vi "Generate Trajectory.vi"(6 "Overrides 2":T1(array[cluster]), 7 "Stoopid Overlap %":dbl min=0.0, 8 "Conditions":T3, 9 "Limits":T2={"Velocity (fps)"=6.0, "Accel (fps^2)"=15.0, "Jerk (fps^3)"=150.0, "StoopidFast (fps)"=6.0} {"StoopidFast (fps)" min=0.0; "Jerk (fps^3)" min=0.0 step=1.0; "Accel (fps^2)" min=0.0; "Velocity (fps)" min=0.0}, 10 "WayPoints":cluster{"x":dbl, "y":dbl, "th":dbl}[](array[cluster]), 11 "Sample Period (s)":dbl=0.02) -> (0 "Updated Waypoints":cluster{"x":dbl, "y":dbl, "th":dbl}[](array[cluster]), 1 "Valid":bool, 2 "Time (s)":dbl, 3 "Trajectory Data":T4(array[cluster]), 4 "Distance (ft)":dbl)   [LabVIEW 2019]
uses:
  Limits.ctl
  Speeds.ctl
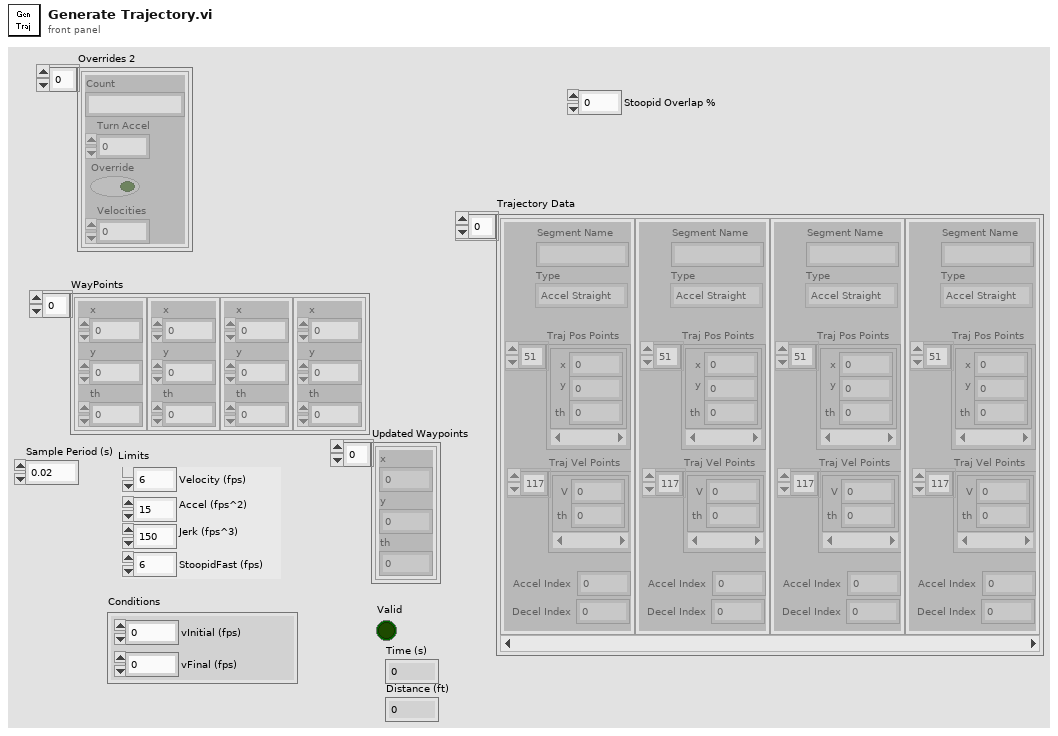
[diagram p1: front panel]
types:
  T1 = cluster{"Count":string, "Turn Accel":dbl, "Override":bool, "Velocities":dbl}[]
  T2 = typedef "Limits.ctl" = cluster{"Velocity (fps)":dbl, "Accel (fps^2)":dbl, "Jerk (fps^3)":dbl, "StoopidFast (fps)":dbl}
  T3 = cluster{"vInitial (fps)":dbl, "vFinal (fps)":dbl}
  T4 = cluster{"Segment Name":string, "Type":enum16{"Accel Straight", "Const Straight", "Blend", "Circle"}, "Traj Pos Points":cluster{"x":dbl, "y":dbl, "th":dbl}[], "Traj Vel Points":cluster{"V":dbl, "th":dbl}[], "Accel Index":i32, "Decel Index":i32}[]
  T5 = typedef "Speeds.ctl" = cluster{"maxV (fps)":dbl, "Accel Limit (fps^2)":dbl, "Initial V (fps)":dbl, "Sample Period (s)":dbl, "Jerk Limit (fps^3)":dbl, "Distances":cluster{"distance (ft)":dbl, "baseline (ft)":dbl, "high (ft)":dbl}[]}
  T6 = cluster{"Count":string, "Turn Accel":dbl, "Override":bool, "Velocities":dbl}
  T7 = cluster{"Point Out":cluster{"x":dbl, "y":dbl, "th":dbl}, "Point Out":cluster{"x":dbl, "y":dbl, "th":dbl}, "Valid":bool}[]
  T8 = typedef "BlendType.ctl" = cluster{"Scaling":dbl, "Length":dbl, "Angle":dbl, "Vertex Dist":dbl, "ParaTime":dbl, "ExtraArc":dbl, "Center Point":cluster{dbl, dbl}, "Radius":dbl}
  T9 = cluster{"Segment Name":string, "Type":enum16{"Accel Straight", "Const Straight", "Blend", "Circle"}, "Traj Pos Points":cluster{"x":dbl, "y":dbl, "th":dbl}[], "Traj Vel Points":cluster{"V":dbl, "th":dbl}[], "Accel Index":i32, "Decel Index":i32}
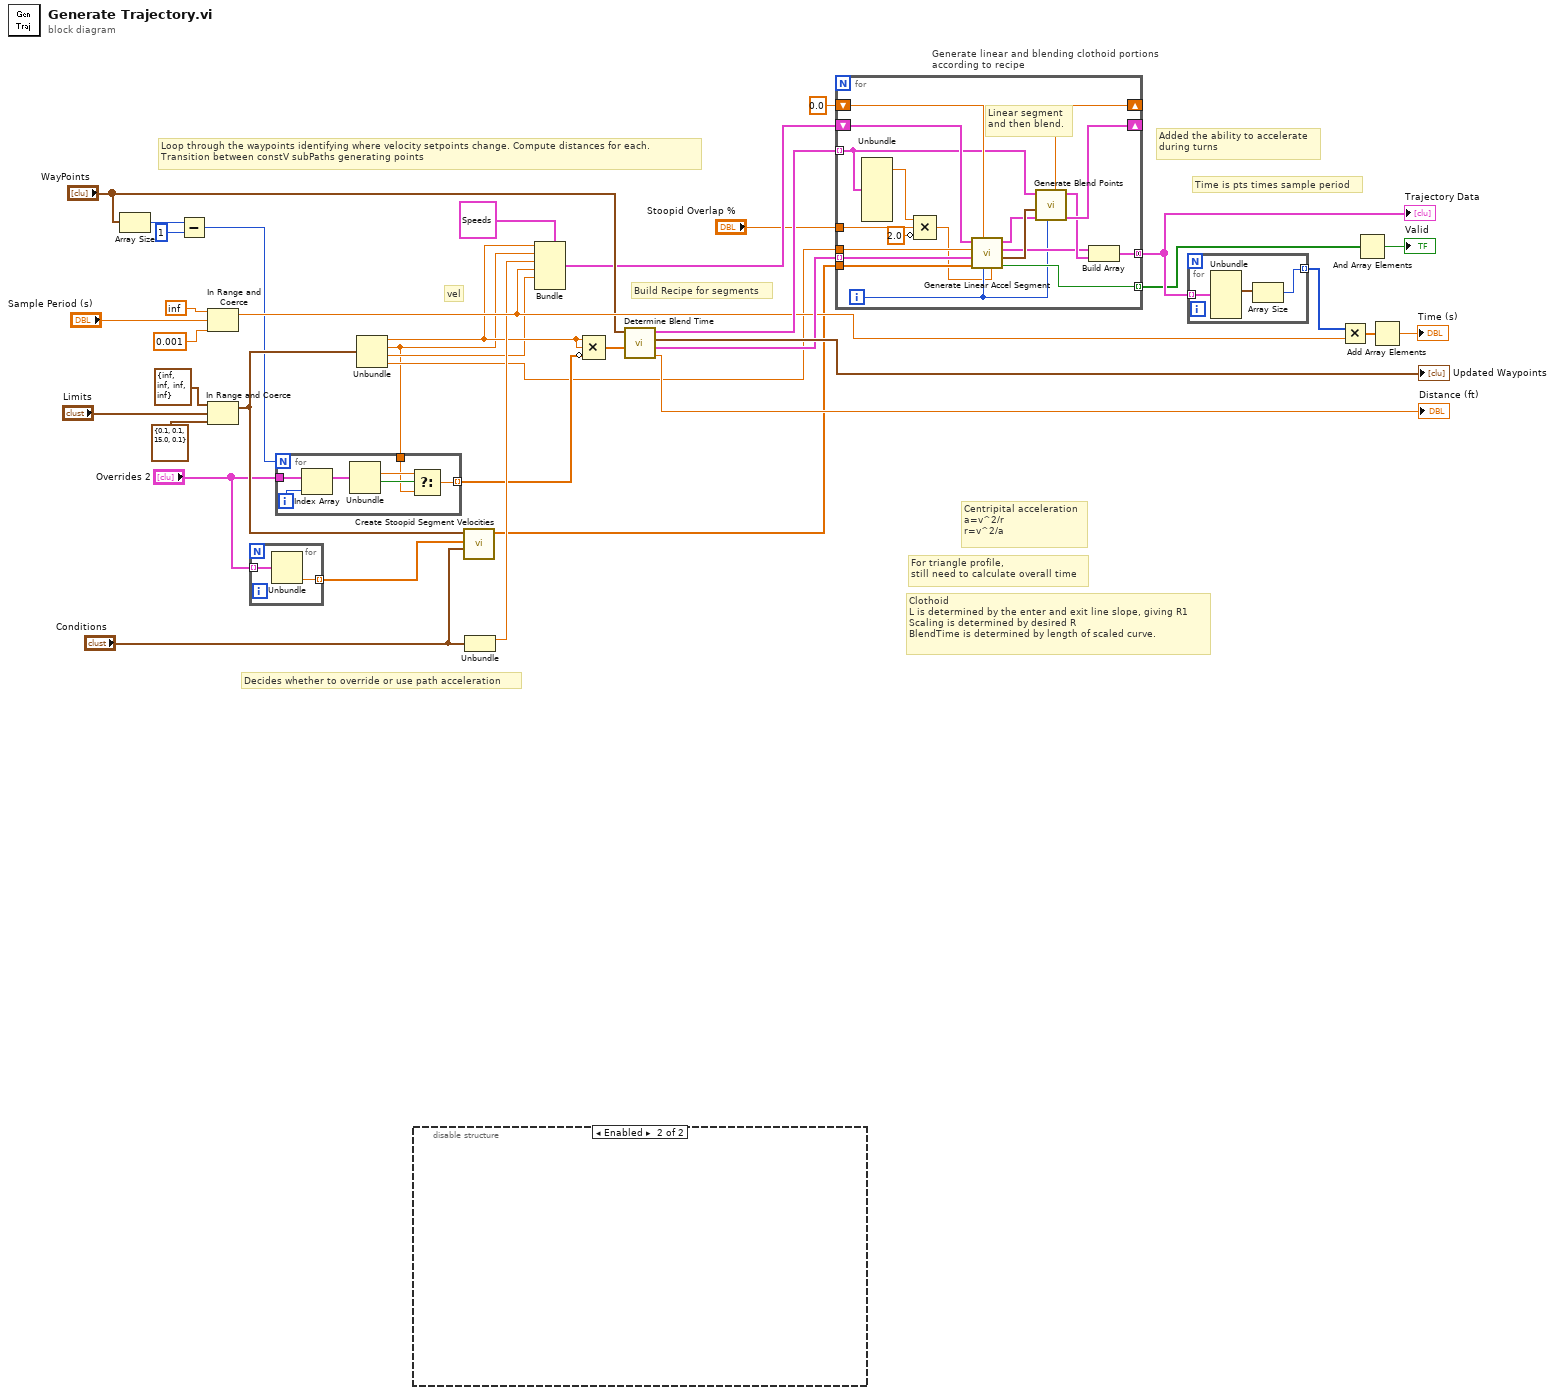
[diagram p0: block diagram]
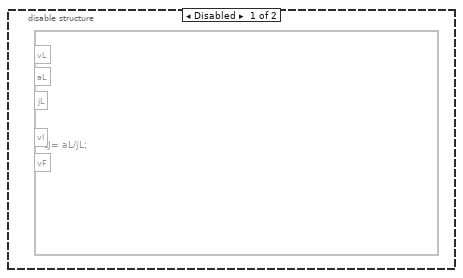
[diagram p2: hidden frame]
diagram:
  # "Loop through the waypoints identifying where velocity setpoints change. Compute distances for each.\nTransition between constV subPaths generating points"
  # "Added the ability to accelerate\nduring turns"
  # "Decides whether to override or use path acceleration"
  # "For triangle profile,\nstill need to calculate overall time"
  # "Build Recipe for segments"
  # "Time is pts times sample period"
  # "Clothoid\nL is determined by the enter and exit line slope, giving R1\nScaling is determined by desired R\nBlendTime is determined by length of scaled curve."
  # "Centripital acceleration\na=v^2/r\nr=v^2/a"
  # "vel"
  n1 = Array Size(array="WayPoints") -> (size(s)=w7:i32)
  n2 = Subtract(x=w7, y=1) -> (x-y=w8:i32)
  n3 = In Range and Coerce(upper limit=inf, x="Sample Period (s)", lower limit=0.001) -> (coerced(x)=w25:dbl)  [unwired: 1 out]
  n4 = In Range and Coerce(upper limit=T2 {"Velocity (fps)"=inf, "Accel (fps^2)"=inf, "Jerk (fps^3)"=inf, "StoopidFast (fps)"=inf} ("Limits"), x="Limits", lower limit=T2 {"Velocity (fps)"=0.1, "Accel (fps^2)"=0.1, "Jerk (fps^3)"=15.0, "StoopidFast (fps)"=0.1} ("Limits")) -> (coerced(x)=w15:T2)  [unwired: 1 out]
  n5 = for {
    tunnel: "Overrides 2" -> [w38] mode=indexing
    tunnel: [w39] -> w4 mode=indexing
    n6 = Unbundle(w38) -> ("Velocities"=w39:dbl)  [unwired: 3 out]
  }
  n7 = Unbundle(w15) -> ("Velocity (fps)"=w21:dbl, "Accel (fps^2)"=w1:dbl, "Jerk (fps^3)"=w2:dbl, "StoopidFast (fps)"=w3:dbl)
  n8 = for {
    N: w8 -> [_]
    tunnel: "Overrides 2" -> [w46]
    tunnel: w1 -> [w43]
    tunnel: [w42] -> w9 mode=indexing
    i -> [w40]
    n9 = Index Array(array=w46, index=w40) -> (element=w41:T6)
    n10 = Unbundle(w41) -> ("Turn Accel"=w44:dbl, "Override"=w45:bool)  [unwired: 2 out]
    n11 = Select(t=w44, s=w45, f=w43) -> (s? t:f=w42:dbl)
  }
  n12 = disable-structure shown="Enabled" {
    frame Disabled {
      n13 = formula code="tJ= aL/jL;"() -> ()  [unwired: 5 in]
    }
    frame Enabled {
    }
  }
  n14 = call "Create Stoopid Segment Velocities.vi"("Conditions"="Conditions", "Velocities"=w4, "Limits"=w15) -> ("Velocities"=w14:dbl[])  [unwired: 8 in]
  n15 = Unbundle("Conditions") -> ("vInitial (fps)"=w23:dbl)  [unwired: 1 out]
  n16 = Bundle(cluster=T5 {"maxV (fps)"=6.0, "Accel Limit (fps^2)"=15.0, "Initial V (fps)"=5.999999999999998, "Sample Period (s)"=0.02, "Jerk Limit (fps^3)"=150.0, "Distances"=[{"distance (ft)"=0.0, "baseline (ft)"=0.0, "high (ft)"=0.0}, {"distance (ft)"=0.3647338133499236, "baseline (ft)"=1.8397338133499224, "high (ft)"=0.9397338133499229}]} ("Speeds in"), "maxV (fps)"=w21, "Accel Limit (fps^2)"=w1, "Initial V (fps)"=w23, "Sample Period (s)"=w25, "Jerk Limit (fps^3)"=w2) -> (w13:T5)  [unwired: 1 in]
  n17 = Compound Arithmetic op=MULTIPLY(w21, w21, invert w9) -> (w20:dbl[])
  n18 = call "Determine Blend Time.vi"("Min R"=w20, "WayPoints"="WayPoints") -> ("Distance"=→"Distance (ft)":dbl, "Linear Info"=w34:T7, "Updated Waypoints"=→"Updated Waypoints":cluster{"x":dbl, "y":dbl, "th":dbl}[], "Blends"=w33:T8[])  [unwired: 6 in]
  n19 = for "Generate linear and blending clothoid portions\naccording to recipe" {
    tunnel: [w65] -> w30 mode=concatenating
    tunnel: w33 -> [w51] mode=indexing
    shift-right: [w64] -> _
    shift-left: w13 -> [w53]
    tunnel: w34 -> [w59] mode=indexing
    tunnel: [w58] -> w28 mode=indexing
    shift-right: [w57] -> _
    shift-left: 0.0 ("Final Acceleration") -> [w56]
    tunnel: w14 -> [w54]
    tunnel: w3 -> [w52]
    tunnel: "Stoopid Overlap %" -> [w49]
    i -> [w55]
    # "Linear segment\nand then blend."
    n20 = Unbundle(w51) -> ("Length"=w50:dbl)  [unwired: 7 out]
    n21 = Compound Arithmetic op=MULTIPLY(w50, w49, invert 2.0 ("value")) -> (w47:dbl)
    n22 = call "Generate Linear Accel Segment.vi"("Stoopid Overlap distance"=w47, "Index"=w55, "Initial Acceleration"=w56, "Velocities"=w54, "Linear Info"=w59, "Stoopid V"=w52, "Speeds in"=w53) -> ("Valid"=w58:bool, "Final Position"=w63:cluster{dbl, dbl, dbl}, "Trajectory Segment"=w61:T9, "Speeds out"=w60:T5)  [unwired: 1 out]
    n23 = call "Generate Blend Points.vi"("Index"=w55, "Speeds in"=w60, "Initial Point"=w63, "Blend Info"=w51) -> ("Speeds out"=w64:T5, "Trajectory Segment"=w62:T9, "Final Acceleration"=w57:dbl)  [unwired: 5 in]
    n24 = Build Array(w61, w62) -> (w65:T4)
  }
  "Trajectory Data" <- w30
  n25 = for {
    tunnel: w30 -> [w68] mode=indexing
    tunnel: [w67] -> w32 mode=indexing
    n26 = Unbundle(w68) -> ("Traj Pos Points"=w66:cluster{"x":dbl, "y":dbl, "th":dbl}[])  [unwired: 5 out]
    n27 = Array Size(array=w66) -> (size(s)=w67:i32)
  }
  n28 = Multiply(x=w32, y=w25) -> (x*y=w31:dbl[])
  n29 = And Array Elements(Boolean array=w28) -> (logical AND=→"Valid":bool)
  n30 = Add Array Elements(numeric array=w31) -> (sum=→"Time (s)":dbl)
